vi "gateSTS.vi"(5 "Store\nSecond Gate?":bool, 6 "Attributes":string[][](array[string]), 10 "Basename":string) -> (3 "Stop Loop":bool)   [LabVIEW 2021]
uses:
  <userlib>/Nanonis Prog Interface V5/Nanonis Prog Interface.lvlib
panel:
  in  "Tabs":T1(tab)
  in  "Start Gate (V)":dbl
  in  "End Gate (V)":dbl
  in  "Increment Gate (V)":dbl
  in  "Stop":bool
  out "Current Gate Voltage (V)":dbl
  in  "?":bool
  out "HDF5 DATANAME":string
  in  "Store\nLock-in\nParameters?":bool
  in  "Store\nTemperatures?":bool
  in  "Store\nMagnetic Field?":bool
  in  "Zigzag Raster?":bool
  in  "Insert Loop Index\ninto Basename?":bool
  in  "Loop Forever?":bool
  out "Loop Index":i32
  in  "Loop Index Offset":i32=1
  in  "Make .dat files?":bool
  out "Ender":bool
  # "Gate STS"
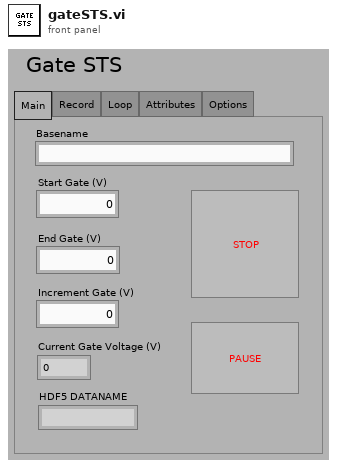
[diagram p1: front panel]
types:
  T1 = enum32{"Main", "Record", "Loop", "Attributes", "Options"}
  T2 = cluster{"Save all":enum16{"no change", "on", "off"}, "Number of Sweeps (0=no change)":i32}
  T3 = enum16{"Set Voltage", "Read Voltage", "Read Current", "Output On", "Output Off", "Set Increment", "Set Increment Time", "Stop Voltage Set", "Set Maximum Voltage", "Get Maximum Voltage"}
  T4 = enum16{"Read State", "Hold", "Ramp to Set", "Ramp to Zero", "Read Switch Heater", "Switch Heater On", "Switch Heater Off", "Read Voltage", "Read Current", "Read Field", "Read Persistent Field", "Read Target Field", "Set Target Field", "Read Ramp Rate", "Set Ramp Rate"}
  T5 = enum16{"pot_temp", "sorb_temp", "needle_valve_temp", "still_temp", "mix_chamber_temp", "stm_rx_temp", "stm_cx_temp", "tank_pressure", "condense_pressure", "still_pressure", "turbo_back_pressure", "n2_trap_pressure"}
  T6 = enum16{"Set Amplitude", "Get Amplitude", "Set Frequency", "Get Frequency", "Set Harmonic", "Get Harmonic", "Set Phase", "Get Phase", "Auto Phase", "Add to Phase", "Autogain", "Set Time Constant", "Get Time Constant", "Set Sensitivity", "Get Sensitivity", "Set Input A", "Set Input A-B", "Get Input Setting", "Set Offset", "Get Offset"}[]
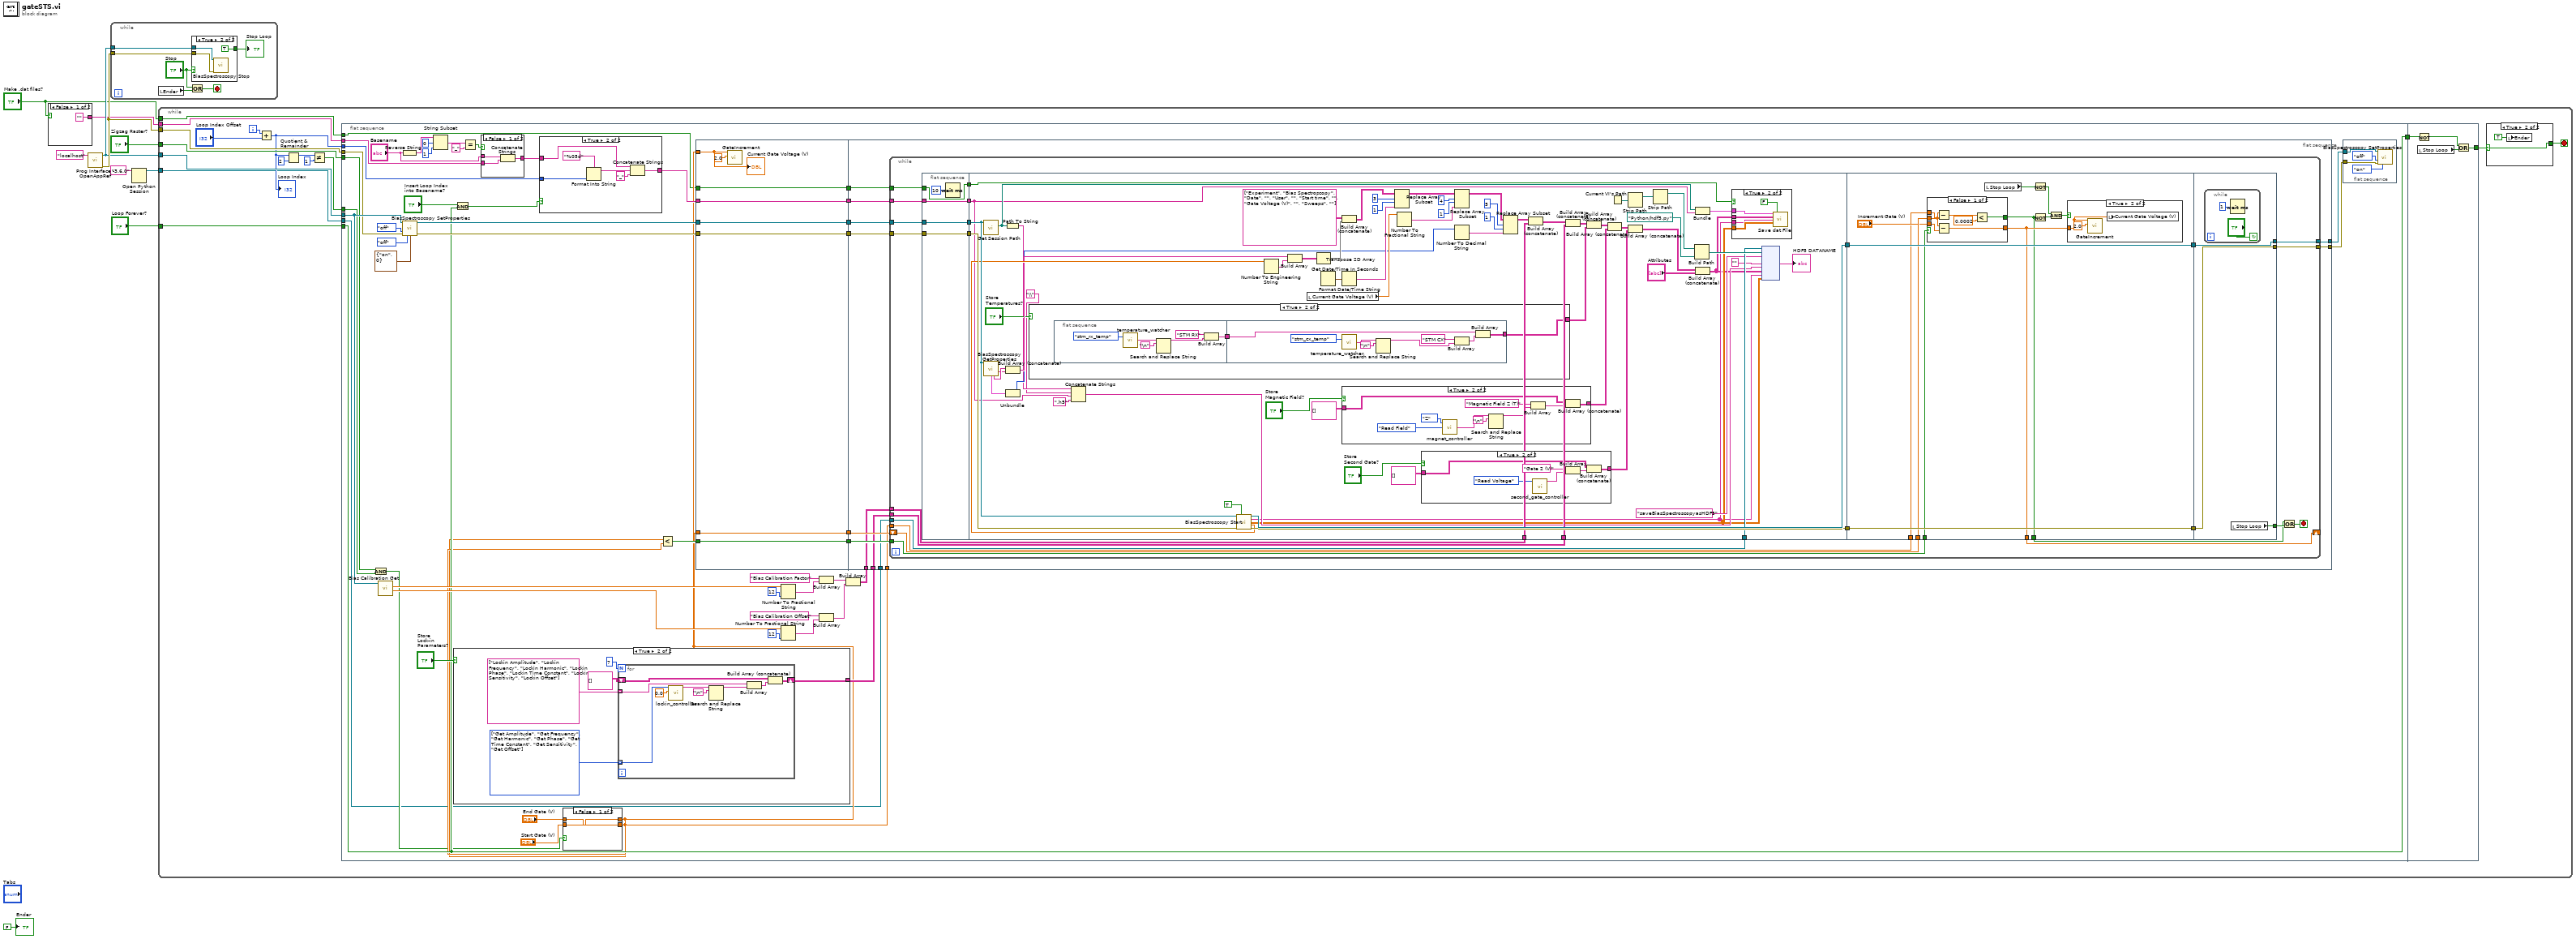
[diagram p0: block diagram]
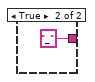
[diagram p2: hidden frame]
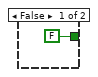
[diagram p3: hidden frame]
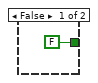
[diagram p4: hidden frame]
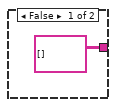
[diagram p8: hidden frame]
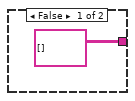
[diagram p12: hidden frame]
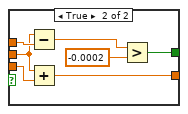
[diagram p13: hidden frame]
diagram:
  n1 = case shown="False" "Make .dat files?" {
    tunnel: ["" ("string") "_" ("string")] -> w2
    frame False {
    }
    frame True {
    }
  }
  n2 = call <userlib>:"Prog Interface - OpenAppRef.vi"("Machine name (local machine IP)"="localhost" ("machine name (localhost)")) -> ("Error out"=w7:errorcluster, "Application reference"=w6:refnum<vi>)  [unwired: 5 in]
  n3 = while {
    tunnel: w6 -> [w18]
    tunnel: w7 -> [w17]
    stop <- w14 stop-if-true
    n4 = local read "Ender"() -> (w13:bool)
    n5 = Or(x="Stop", y=w13) -> (x .or. y?=w14:bool)
    n6 = case shown="True" "Stop" {
      tunnel: w18 -> [_ w22]
      tunnel: w17 -> [_ w21]
      tunnel: [FALSE TRUE] -> w16
      frame False {
      }
      frame True {
        n7 = call <userlib>:"BiasSpectroscopy Stop.vi"("Application ref in"=w22, "Error in (no error)"=w21) -> ()  [unwired: 12 in, 2 out]
      }
    }
    "Stop Loop" <- w16
  }
  n8 = Open Python Session(python version="3.6.0" ("Python version")) -> (session out=w4:refnum<k35>)  [unwired: 2 in, 1 out]
  n9 = while {
    tunnel: "Loop Forever?" -> [w39]
    tunnel: w6 -> [w37]
    tunnel: w7 -> [w36]
    tunnel: "Zigzag Raster?" -> [w32]
    tunnel: w4 -> [w25]
    tunnel: w2 -> [w24]
    tunnel: "Make .dat files?" -> [w23]
    i -> [w33]
    stop <- w34 stop-if-true
    n10 = Add(x=w33, y="Loop Index Offset") -> (x+y=w30:i32)
    "Loop Index" <- w30
    n11 = Quotient & Remainder(x=w30, y=2) -> (x-y*floor(x/y)=w28:i32)  [unwired: 1 out]
    n12 = Not Equal?(x=w28, y=1) -> (x != y?=w26:bool)
    n13 = flat-sequence {
      tunnel: w39 -> [w64]
      tunnel: [w64] -> w38
      tunnel: w37 -> [w68]
      tunnel: w36 -> [w67]
      tunnel: w30 -> [w62]
      tunnel: w32 -> [w49]
      tunnel: w26 -> [w48]
      tunnel: w25 -> [w46]
      tunnel: w24 -> [w45]
      tunnel: w23 -> [w43]
      tunnel: w38 -> [w319]
      tunnel: [w316] -> w35
      frame #0 {
        n14 = And(x=w49, y=w48) -> (x .and. y?=w47:bool)
        n15 = call <userlib>:"Bias Calibration Get.vi"("Application ref in"=w68) -> ("Offset (V)"=w78:sgl, "Calibration (V/V)"=w79:sgl)  [unwired: 7 in, 2 out]
        n16 = Reverse String(1:"Basename") -> (0:w59:string)
        n17 = call <userlib>:"BiasSpectroscopy SetProperties.vi"("Application ref in"=w68, "Autosave (no change)"=enum16{"no change", "on", "off"}."off", "Error in (no error)"=w67, "Save dialog"=enum16{"no change", "on", "off"}."off", "Multiple sweeps config"=T2 {"Save all"=enum."on", "Number of Sweeps (0=no change)"=0}) -> ("Application ref out"=w88:refnum<vi>, "Error out"=w89:errorcluster)  [unwired: 9 in]
        n18 = String Subset(string=w59, offset (0)=0, length (rest)=1 ("length (rest)")) -> (substring=w58:string)
        n19 = case shown="True" "Store\nLock-in\nParameters?" {
          tunnel: [string[][] [] w111] -> w80
          frame False {
          }
          frame True {
            w114 = T6 [enum."Get Amplitude", enum."Get Frequency", enum."Get Harmonic", enum."Get Phase", enum."Get Time Constant", enum."Get Sensitivity", enum."Get Offset"] items=["Set Amplitude", "Get Amplitude", "Set Frequency", "Get Frequency", "Set Harmonic", "Get Harmonic", "Set Phase", "Get Phase", "Auto Phase", "Add to Phase", "Autogain", "Set Time Constant", "Get Time Constant", "Set Sensitivity", "Get Sensitivity", "Set Input A", "Set Input A-B", "Get Input Setting", "Set Offset", "Get Offset"]
            n20 = for {
              N: 7 -> [_]
              tunnel: w114 -> [w122] mode=indexing
              tunnel: string[] ["Lockin Amplitude", "Lockin Frequency", "Lockin Harmonic", "Lockin Phase", "Lockin Time Constant", "Lockin Sensitivity", "Lockin Offset"] -> [w121] mode=indexing
              shift-right: [w119] -> w111
              shift-left: string[][] [] -> [w120]
              n21 = call "lockin_controller.vi"("Numerical Argument"=0.0, "Command"=w122) -> ("Response"=w117:string)  [unwired: 9 in]
              n22 = Search and Replace String(input string=w117, search string="\n") -> (result string=w118:string)  [unwired: 6 in, 3 out]
              n23 = Build Array(w121, w118) -> (w123:string[])
              n24 = Build Array (concatenate)(w120, w123) -> (w119:string[][])
            }
          }
        }
        n25 = And(x="Insert Loop Index\ninto Basename?", y=w64) -> (x .and. y?=w63:bool)
        n26 = Equal?(x=w58, y="_") -> (x = y?=w56:bool)
        n27 = case shown="False" w56 {
          tunnel: "Basename" -> [w101 w102]
          tunnel: [w100 w102] -> w54
          tunnel: w45 -> [w99 _]
          frame False {
            n28 = Concatenate Strings(w101, w99) -> (w100:string)
          }
          frame True {
          }
        }
        n29 = case shown="True" w63 {
          tunnel: [w103 w109] -> w66
          tunnel: w54 -> [w103 w108]
          tunnel: w62 -> [_ w106]
          frame False {
          }
          frame True {
            n30 = Format Into String(format string="%05d", w106) -> (resulting string=w104:string)  [unwired: 2 in, 1 out]
            n31 = Concatenate Strings(w108, w104, "_" ("string")) -> (w109:string)
          }
        }
        n32 = case shown="False" w47 {
          tunnel: "End Gate (V)" -> [w96 w98]
          tunnel: [w96 w97] -> w52
          tunnel: [w95 w98] -> w51
          tunnel: "Start Gate (V)" -> [w95 w97]
          frame False {
          }
          frame True {
          }
        }
        n33 = Less?(x=w51, y=w52) -> (x < y?=w83:bool)
        n34 = flat-sequence {
          tunnel: w51 -> [w132]
          tunnel: w83 -> [w133]
          tunnel: w88 -> [w134]
          tunnel: w89 -> [w135]
          tunnel: w66 -> [w136]
          tunnel: [w136] -> w94
          tunnel: [w135] -> w93
          tunnel: [w134] -> w92
          tunnel: [w133] -> w91
          tunnel: [w132] -> w90
          tunnel: w51 -> [w130]
          tunnel: [w129] -> w44
          tunnel: w43 -> [w129]
          tunnel: [w145] -> w86
          tunnel: [w144] -> w85
          tunnel: w94 -> [w148]
          tunnel: w93 -> [w147]
          tunnel: w92 -> [w146]
          tunnel: w91 -> [w143]
          tunnel: w90 -> [w142]
          tunnel: w52 -> [w141]
          tunnel: w80 -> [w140]
          tunnel: w69 -> [w139]
          tunnel: w46 -> [w138]
          tunnel: w44 -> [w137]
          frame #0 {
            n35 = call "GateIncrement.vi"("Increment"=2.0, "Gate Voltage"=w130) -> ()  [unwired: 10 in]
            "Current Gate Voltage (V)" <- w130
          }
          frame #1 {
            n36 = while {
              tunnel: w148 -> [w172]
              tunnel: w147 -> [w171]
              tunnel: w146 -> [w170]
              tunnel: [w169] -> w145
              tunnel: [w168] -> w144
              tunnel: w143 -> [w154]
              shift-right: [w158] -> _
              shift-left: w142 -> [w156]
              tunnel: w141 -> [w155]
              tunnel: w140 -> [w153]
              tunnel: w139 -> [w152]
              tunnel: w138 -> [w151]
              tunnel: w137 -> [w149]
              stop <- w159 stop-if-true
              n37 = flat-sequence {
                tunnel: w170 -> [w175]
                tunnel: w171 -> [w176]
                tunnel: w172 -> [w177]
                tunnel: [w177] -> w163
                tunnel: [w176] -> w162
                tunnel: [w175] -> w161
                tunnel: [w173] -> w150
                tunnel: w149 -> [w173]
                tunnel: [w241] -> w165
                tunnel: [w242] -> w164
                tunnel: w163 -> [w198]
                tunnel: w162 -> [w243]
                tunnel: w161 -> [w239]
                tunnel: w153 -> [w214]
                tunnel: w152 -> [w212]
                tunnel: w151 -> [w201]
                tunnel: w150 -> [w187]
                tunnel: [w294] -> w167
                tunnel: [w293] -> w166
                tunnel: w165 -> [w294]
                tunnel: w164 -> [w293]
                tunnel: [w289] -> w158
                tunnel: [w287] -> w157
                tunnel: w156 -> [w286]
                tunnel: w155 -> [w284]
                tunnel: w154 -> [w283]
                tunnel: [w312] -> w169
                tunnel: [w313] -> w168
                tunnel: w167 -> [w313]
                tunnel: w166 -> [w312]
                tunnel: [w311] -> w160
                frame #0 {
                  n38 = Wait (ms)(milliseconds to wait=u32 10) -> ()  [unwired: 1 out]
                }
                frame #1 {
                  n39 = call <userlib>:"Get Session Path.vi"("Application ref in"=w239) -> ("Session path"=w199:path)  [unwired: 8 in, 2 out]
                  n40 = call <userlib>:"BiasSpectroscopy GetProperties.vi"("Application ref in"=w239) -> ("Parameters"=w231:string[], "Multiple sweeps configuration"=w220:cluster{"Number of Sweeps":i32, "Save all":bool}, "Fixed parameters"=w232:string[])  [unwired: 7 in, 5 out]
                  n41 = Unbundle(w220) -> ("Number of Sweeps"=w219:i32)  [unwired: 1 out]
                  n42 = Path To String(path=w199) -> (string=w192:string)
                  n43 = Build Array (concatenate)(w232, w231) -> (w236:string[])
                  n44 = case shown="True" "Store\nTemperatures?" {
                    tunnel: [string[][] [] w267] -> w208
                    frame False {
                    }
                    frame True {
                      n45 = flat-sequence {
                        tunnel: [w272] -> w268
                        tunnel: w268 -> [w279]
                        tunnel: [w278] -> w267
                        frame #0 {
                          n46 = call "temperature_watcher.vi"("Command"=T5."stm_rx_temp") -> ("Response"=w270:string)  [unwired: 1 in]
                          n47 = Search and Replace String(input string=w270, search string="\n") -> (result string=w269:string)  [unwired: 6 in, 3 out]
                          n48 = Build Array("STM RX" ("element"), w269) -> (w272:string[])
                        }
                        frame #1 {
                          n49 = call "temperature_watcher.vi"("Command"=T5."stm_cx_temp") -> ("Response"=w276:string)  [unwired: 1 in]
                          n50 = Search and Replace String(input string=w276, search string="\n") -> (result string=w275:string)  [unwired: 6 in, 3 out]
                          n51 = Build Array("STM CX" ("element"), w275) -> (w280:string[])
                          n52 = Build Array(w279, w280) -> (w278:string[][])
                        }
                      }
                    }
                  }
                  n53 = Concatenate Strings(w192, "\\" ("string"), w198, ".h5" ("string")) -> (w196:string)
                  n54 = call <userlib>:"BiasSpectroscopy Start.vi"("Application ref in"=w239, "Get data (F)"=TRUE, "Error in (no error)"=w243) -> ("Application ref out"=w242:refnum<vi>, "Channels"=w189:string[], "Data"=w190:sgl[][], "Parameters"=w238:sgl[], "Error out"=w241:errorcluster)  [unwired: 8 in]
                  n55 = Number To Engineering String(4:w238) -> (0:w237:string[])  [unwired: 3 in]
                  n56 = Build Array(w236, w237) -> (w235:string[][])
                  n57 = local read "Current Gate Voltage (V)"() -> (w222:dbl)
                  n58 = Transpose 2D Array(2D array=w235) -> (transposed array=w233:string[][])
                  n59 = Get Date/Time In Seconds() -> (seconds since 1Jan1904=w230:timestamp)
                  n60 = Build Array (concatenate)(string[][] [["Experiment", "Bias Spectroscopy"], ["Date", ""], ["User", ""], ["Start time", ""], ["Gate Voltage (V)", ""], ["Sweeps", ""]] ("Attributes"), w233) -> (w229:string[][])
                  n61 = Format Date/Time String(seconds (now)=w230) -> (date/time string=w228:string)  [unwired: 2 in]
                  n62 = case shown="True" "Store\nMagnetic Field?" {
                    tunnel: [w256 w260] -> w205
                    tunnel: string[][] [] ("array") -> [w256 w261]
                    frame False {
                    }
                    frame True {
                      n63 = call "magnet_controller.vi"("Command"=T4."Read Field", "Direction"=enum16{"X", "Y", "Z"}."Z") -> ("Response"=w258:string)  [unwired: 1 in]
                      n64 = Search and Replace String(input string=w258, search string="\n") -> (result string=w257:string)  [unwired: 6 in, 3 out]
                      n65 = Build Array("Magnetic Field Z (T)" ("element"), w257) -> (w262:string[])
                      n66 = Build Array (concatenate)(w261, w262) -> (w260:string[][])
                    }
                  }
                  n67 = Replace Array Subset(array=w229, new element=w228, index (row)=3, index (col)=1 ("disabled index (col)")) -> (w225:string[][])
                  n68 = Number To Fractional String(number=w222) -> (F-format string=w221:string)  [unwired: 3 in]
                  n69 = case shown="True" "Store\nSecond Gate?" {
                    tunnel: [w244 w247] -> w178
                    tunnel: string[][] [] ("array") -> [w244 w248]
                    frame False {
                    }
                    frame True {
                      n70 = call "second_gate_controller.vi"("Command"=T3."Read Voltage") -> ("Response"=w246:string)  [unwired: 10 in]
                      n71 = Build Array("Gate 2 (V)" ("element"), w246) -> (w249:string[])
                      n72 = Build Array (concatenate)(w248, w249) -> (w247:string[][])
                    }
                  }
                  n73 = Replace Array Subset(array=w225, new element=w221, index (row)=4, index (col)=1 ("disabled index (col)")) -> (w218:string[][])
                  n74 = Number To Decimal String(number=w219) -> (decimal integer string=w215:string)  [unwired: 1 in]
                  n75 = Replace Array Subset(array=w218, new element=w215, index (row)=5, index (col)=1 ("disabled index (col)")) -> (w213:string[][])
                  n76 = Build Array (concatenate)(w213, w212) -> (w211:string[][])
                  n77 = Build Array (concatenate)(w211, w214) -> (w209:string[][])
                  n78 = Build Array (concatenate)(w209, w208) -> (w206:string[][])
                  n79 = Build Array (concatenate)(w206, w205) -> (w182:string[][])
                  n80 = Current VI's Path() -> (path=w193:path)
                  n81 = Strip Path(path=w193) -> (stripped path=w194:path)  [unwired: 1 out]
                  n82 = Build Array (concatenate)(w182, w178) -> (w181:string[][])
                  n83 = Strip Path(path=w194) -> (stripped path=w195:path)  [unwired: 1 out]
                  n84 = Build Path(base path=w195, name or relative path=path "Python/hdf5.py") -> (appended path=w202:path)
                  n85 = Bundle("Session path"=w199, "Basename"=w198) -> (w188:cluster{"Session path":path, "Basename":string})  [unwired: 1 in]
                  n86 = Build Array (concatenate)(w181, "Attributes") -> (w183:string[][])
                  n87 = case shown="True" w187 {
                    tunnel: w183 -> [_ w255]
                    tunnel: w190 -> [_ w254]
                    tunnel: w189 -> [_ w253]
                    tunnel: w188 -> [_ w252]
                    frame False {
                    }
                    frame True {
                      n88 = call <userlib>:"Save dat File.vi"("Filename control"=w252, "Show save dialog (T)"=FALSE, "Attributes"=w255, "Channels names"=w253, "Data"=w254) -> ()  [unwired: 7 in, 4 out]
                    }
                  }
                  n89 = node(w201, w202, "saveBiasSpectroscopyasHDF5" ("function name"), "" ("function name"), w196, w183, w189, w190) -> (→"HDF5 DATANAME":string)  [unwired: 5 in, 4 out]
                }
                frame #2 {
                  n90 = case shown="False" w283 {
                    tunnel: w286 -> [w299 w305]
                    tunnel: "Increment Gate (V)" -> [w300 w308]
                    tunnel: [w301 w307] -> w289
                    tunnel: w284 -> [w298 w306]
                    tunnel: [w296 w304] -> w287
                    frame False {
                      n91 = Subtract(x=w299, y=w298) -> (x-y=w297:dbl)
                      n92 = Subtract(x=w299, y=w300) -> (x-y=w301:dbl)
                      n93 = Less?(x=w297, y=0.0002) -> (x < y?=w296:bool)
                    }
                    frame True {
                      n94 = Subtract(x=w305, y=w306) -> (x-y=w303:dbl)
                      n95 = Add(x=w305, y=w308) -> (x+y=w307:dbl)
                      n96 = Greater?(x=w303, y=-0.0002) -> (0:w304:bool)
                    }
                  }
                  n97 = local read "Stop Loop"() -> (w292:bool)
                  n98 = Not(x=w292) -> (.not. x?=w290:bool)
                  n99 = Not(x=w287) -> (.not. x?=w288:bool)
                  n100 = And(x=w290, y=w288) -> (x .and. y?=w291:bool)
                  n101 = case shown="True" w291 {
                    tunnel: w289 -> [_ w310]
                    frame False {
                    }
                    frame True {
                      n102 = call "GateIncrement.vi"("Increment"=2.0, "Gate Voltage"=w310) -> ()  [unwired: 10 in]
                      n103 = local write "Current Gate Voltage (V)"(w310) -> ()
                    }
                  }
                }
                frame #3 {
                  n104 = while {
                    stop <- "?" continue-if-true
                    n105 = Wait (ms)(milliseconds to wait=u32 1) -> ()  [unwired: 1 out]
                  }
                  n106 = local read "Stop Loop"() -> (w311:bool)
                }
              }
              n107 = Or(x=w157, y=w160) -> (x .or. y?=w159:bool)
            }
          }
        }
        n108 = Number To Fractional String(number=w79, precision (6)=i16 12) -> (F-format string=w75:string)  [unwired: 2 in]
        n109 = Number To Fractional String(number=w78, precision (6)=i16 12) -> (F-format string=w72:string)  [unwired: 2 in]
        n110 = Build Array("Bias Calibration Factor" ("element"), w75) -> (w70:string[])
        n111 = Build Array("Bias Calibration Offset" ("element"), w72) -> (w71:string[])
        n112 = Build Array(w70, w71) -> (w69:string[][])
        n113 = flat-sequence {
          tunnel: w86 -> [w128]
          tunnel: w85 -> [w127]
          frame #0 {
            n114 = call <userlib>:"BiasSpectroscopy SetProperties.vi"("Application ref in"=w128, "Autosave (no change)"=enum16{"no change", "on", "off"}."off", "Error in (no error)"=w127, "Save dialog"=enum16{"no change", "on", "off"}."on") -> ()  [unwired: 10 in, 2 out]
          }
        }
      }
      frame #1 {
        n115 = Not(x=w319) -> (.not. x?=w317:bool)
        n116 = local read "Stop Loop"() -> (w318:bool)
        n117 = Or(x=w317, y=w318) -> (x .or. y?=w316:bool)
      }
    }
    n118 = case shown="True" w35 {
      selector: w35 -> [_ w42]
      tunnel: [FALSE w42] -> w34
      frame False {
      }
      frame True {
        n119 = local write "Ender"(TRUE ("Ender")) -> ()
      }
    }
  }
  "Ender" <- FALSE ("Ender")
